vi "Impedance tube v0.7.vi"() -> ()   [LabVIEW 2021]
uses:
  <vilib>/express/express analysis/Spectral/Block/exnSpectralBlock spectral measurements RMS poly.vi
  <vilib>/express/express analysis/Spectral/Block/exnSpectralBlock spectral measurements RMS DDT.vi
  <vilib>/express/express arith-compare/Formula/XNode/ExpressFormulaBlockNode.xnode
  <vilib>/express/express analysis/Spectral/XNode/ExpressSpectralMeasurementsBlockNode.xnode
  <vilib>/ptbypt/NI_PtbyPt.lvlib
  <vilib>/Analysis/NI_AALPro.lvlib
panel:
  out "Probe":dbl[](graph)
  out "Rr":dbl[](graph)
  out "Absorption coeff":dbl[](graph)
  in  "number of samples":i32=2048
  out "MIC 2":dynamicdata(graph)
  out "FFT2":dynamicdata(graph)
  out "MIC 2":dbl
  out "FFT1":dynamicdata(graph)
  out "MIC 1":dynamicdata(graph)
  out "MIC 1":dbl
  in  "stop (F)":bool
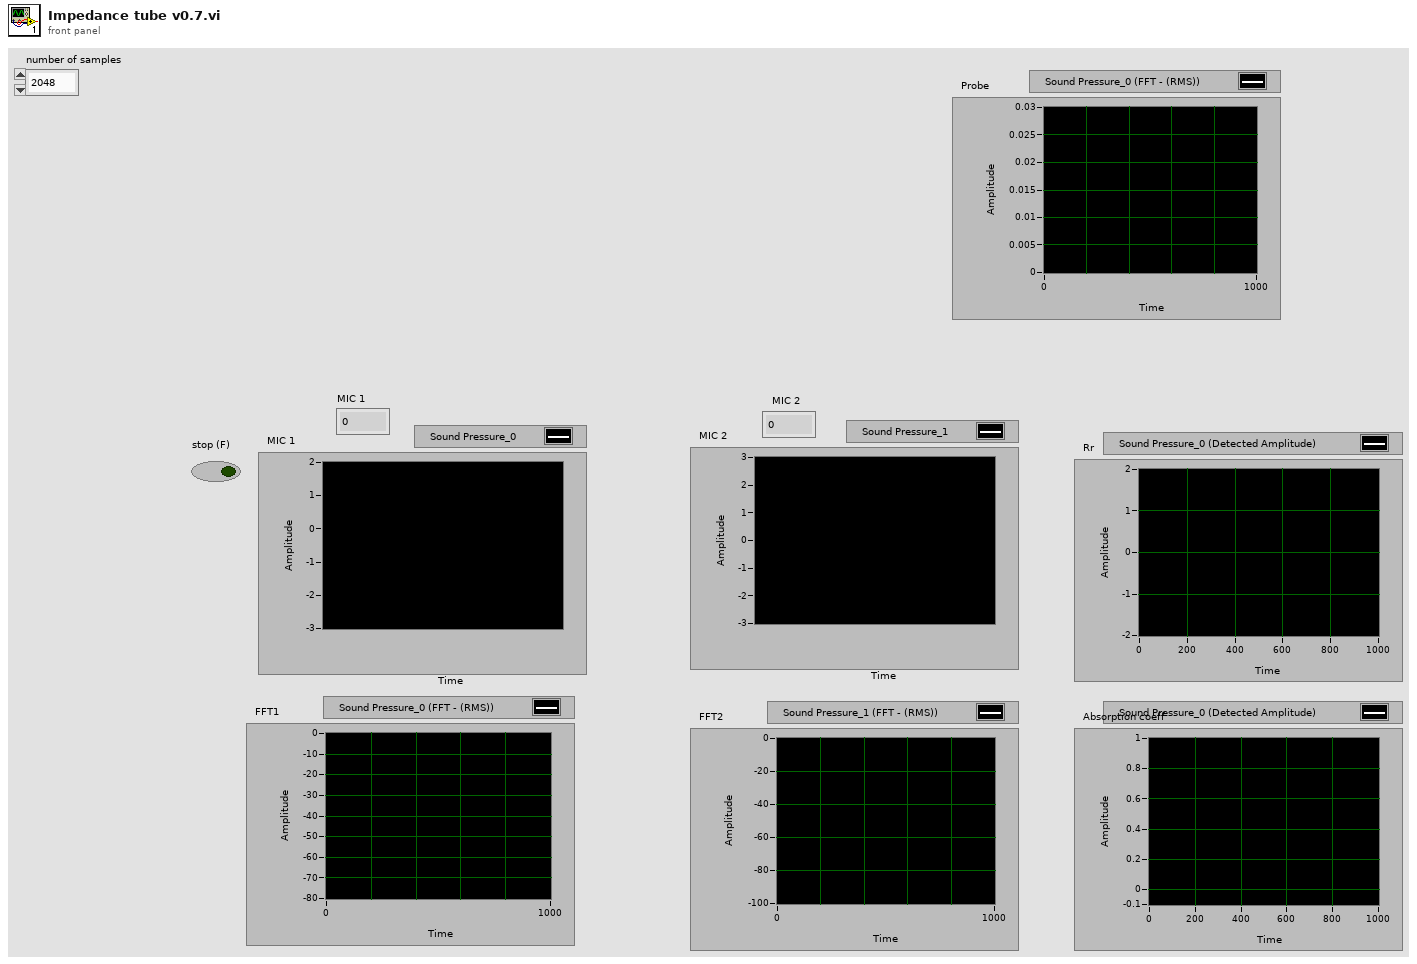
[diagram p1: front panel]
types:
  T1 = cluster{"averaging mode":u16, "weighting mode":u16, "number of averages":u32}
  T2 = cluster{"dB On (F)":bool, "unwrap phase (F)":bool, "convert to degree (F)":bool}
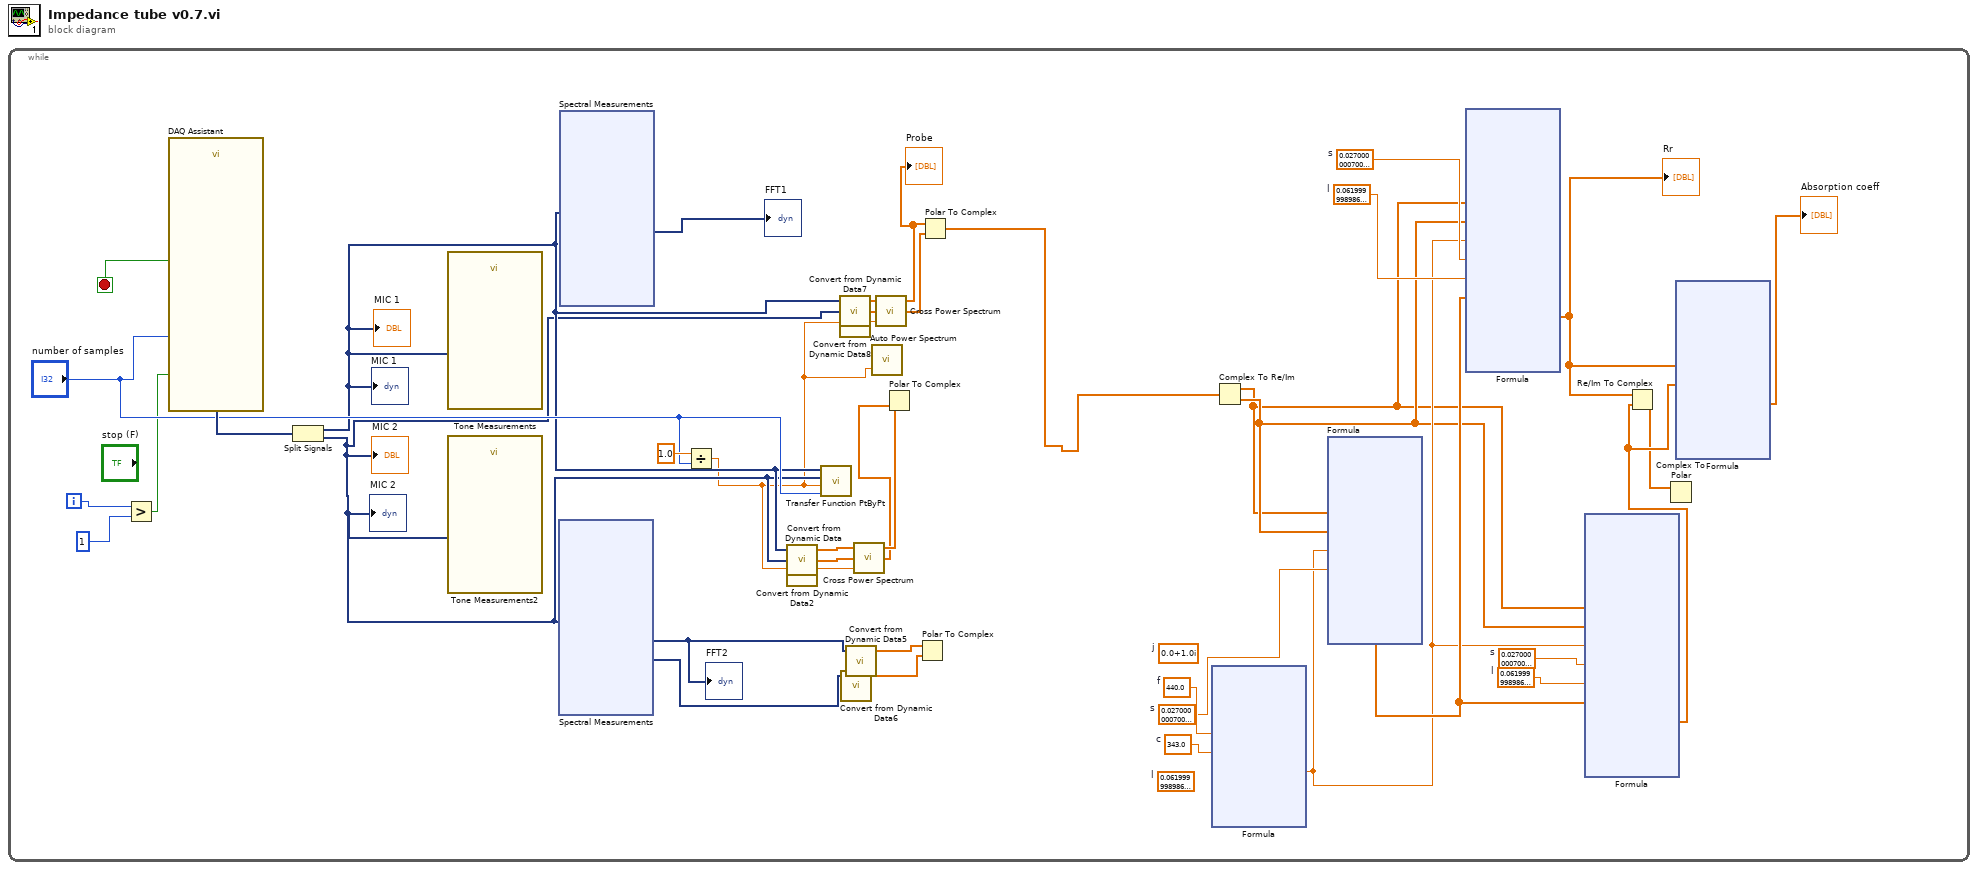
[diagram p0: block diagram]
diagram:
  n1 = while {
    i -> [w26]
    stop <- w39 stop-if-true
    w31 = sgl 0.062  # l
    w32 = sgl 0.027  # s
    w33 = sgl 0.062  # l
    w34 = sgl 0.027  # s
    (unwired) sgl 0.062  # l
    w37 = sgl 440.0  # f
    w35 = sgl 0.027  # s
    w36 = sgl 343.0  # c
    (unwired) csg 0.0+1.0i  # j
    n2 = Greater?(x=w26, y=1) -> (0:w14:bool)
    n3 = call "DAQ Assistant"("number of samples"="number of samples", "stop (F)"=w14) -> ("data"=w38:dynamicdata, "stopped"=w39:bool)  [unwired: 14 in, 2 out]
    n4 = Split Signals(w38) -> (w8:dynamicdata, w6:dynamicdata)  [unwired: 2 in]
    "MIC 1" <- w8
    "MIC 1" <- w8
    "MIC 2" <- w6
    "MIC 2" <- w6
    n5 = call "Tone Measurements"("Signals"=w8) -> ()  [unwired: 8 in, 3 out]
    n6 = call "Tone Measurements2"("Signals"=w6) -> ()  [unwired: 8 in, 3 out]
    n7 = xnode "Spectral Measurements"("Signals"=w6) -> ("FFT - (RMS)"=w10:dynamicdata, "Phase"=w9:dynamicdata)  [unwired: 1 in, 1 out]
    "FFT2" <- w10
    n8 = xnode "Spectral Measurements"("Signals"=w8) -> ("FFT - (RMS)"=→"FFT1":dynamicdata)  [unwired: 1 in, 2 out]
    n9 = Divide(x=1.0, y="number of samples") -> (x/y=w3:dbl)
    n10 = call "Convert from Dynamic Data"("Dynamic Data Type"=w8) -> ("Array"=w18:dbl[])  [unwired: 3 in]
    n11 = call "Convert from Dynamic Data2"("Dynamic Data Type"=w6) -> ("Array"=w17:dbl[])  [unwired: 3 in]
    n12 = call <vilib>:"Transfer Function PtByPt.vi"("sample length"="number of samples", "dt"=w3, "response signal y"=w6, "stimulus signal x"=w8) -> ()  [unwired: 1 in, 4 out]
    n13 = call "Convert from Dynamic Data7"("Dynamic Data Type"=w8) -> ("Array"=w7:dbl[])  [unwired: 3 in]
    n14 = call "Convert from Dynamic Data8"("Dynamic Data Type"=w6) -> ("Array"=w5:dbl[])  [unwired: 3 in]
    n15 = call "Convert from Dynamic Data6"("Dynamic Data Type"=w9) -> ("Array"=w12:dbl[])  [unwired: 3 in]
    n16 = call "Convert from Dynamic Data5"("Dynamic Data Type"=w10) -> ("Array"=w11:dbl[])  [unwired: 3 in]
    n17 = call <vilib>:"Cross Power Spectrum.vi"("dt"=w3, "Signal Y (V)"=w17, "Signal X (V)"=w18) -> ("Cross Power XY Spectrum Phase (radians)"=w15:dbl[], "Cross Power XY Spectrum Mag (V^2rms)"=w16:dbl[])  [unwired: 1 out]
    n18 = call <vilib>:"Auto Power Spectrum.vi"("dt"=w3) -> ()  [unwired: 1 in, 2 out]
    n19 = call <vilib>:"Cross Power Spectrum.vi"("dt"=w3, "Signal Y (V)"=w5, "Signal X (V)"=w7) -> ("Cross Power XY Spectrum Phase (radians)"=w4:dbl[], "Cross Power XY Spectrum Mag (V^2rms)"=w2:dbl[])  [unwired: 1 out]
    "Probe" <- w2
    n20 = Polar To Complex(1:w15, 2:w16) -> ()  [unwired: 1 out]
    n21 = Polar To Complex(1:w12, 2:w11) -> ()  [unwired: 1 out]
    n22 = Polar To Complex(1:w4, 2:w2) -> (0:w1:cdb[])
    n23 = xnode "Formula"("f"=w37, "c"=w36) -> ("Result"=w29:sgl)  [unwired: 1 in, 1 out]
    n24 = Complex To Re/Im(x + iy=w1) -> (x=w23:dbl[], y=w28:dbl[])
    n25 = xnode "Formula"("Hr"=w23, "Hi"=w28, "k"=w29, "s"=w35) -> ("Result"=w30:dbl[])  [unwired: 1 in, 1 out]
    n26 = xnode "Formula"("Hr"=w23, "Hi"=w28, "k"=w29, "s"=w34, "l"=w33, "D"=w30) -> ("Result"=w19:dbl[])  [unwired: 1 in, 1 out]
    "Rr" <- w19
    n27 = xnode "Formula"("Hr"=w23, "Hi"=w28, "k"=w29, "s"=w32, "l"=w31, "D"=w30) -> ("Result"=w27:dbl[])  [unwired: 1 in, 1 out]
    n28 = Re/Im To Complex(1:w27, 2:w19) -> (0:w24:cdb[])
    n29 = Complex To Polar(r * e^(i*theta)=w24) -> ()  [unwired: 2 out]
    n30 = xnode "Formula"("Rr"=w19, "Ri"=w27) -> ("Result"=→"Absorption coeff":dbl[])  [unwired: 1 in, 1 out]
  }
